vi "Initialize Virtual Microscope.vi"(8 "error in (no error)":errorcluster, 11 "Application in":refnum<class "Application.lvclass">) -> (0 "error out":errorcluster, 3 "Application out":refnum<class "Application.lvclass">)   [LabVIEW 2023, in "Application.lvlib" / "Application.lvclass"]
uses:
  Application.lvclass
  Application.lvclass/Application.ctl
  <vilib>/ActorFramework/Actor/Actor.lvclass
  User Interface/Splash Screen Messages/Update Status Msg/Update Status Msg.lvclass
  Hardware/Microscope/Microscope.lvclass
  C:/FlashGordon/Development/Hardware/Device/Device.lvclass
  C:/Program Files/National Instruments/LabVIEW 2023/vi.lib/ActorFramework/Actor/Actor.lvclass
  C:/FlashGordon/Development/Hardware/Microscope/Microscope.lvclass
  C:/FlashGordon/Development/Application/Application.lvclass
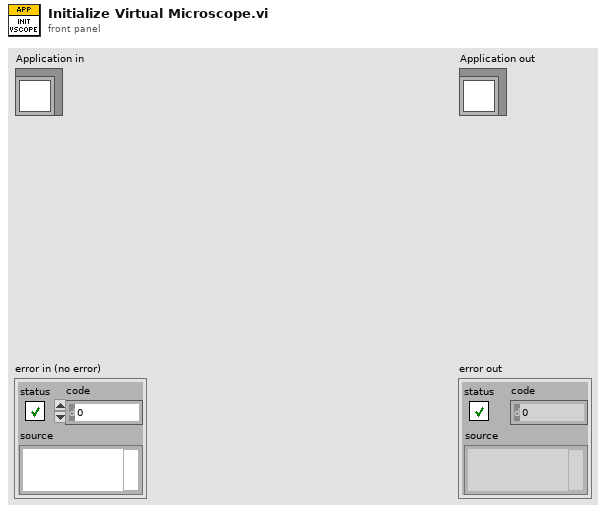
[diagram p1: front panel]
types:
  T1 = typedef "Microscope Type.ctl" = enum16{"Disable", "TE2000", "Eclipse Ti", "Ti2"}
  T2 = typedef "Microscope Configuration.ctl" = cluster{"Serial Port":refnum<visa-resource-name>, "Microscope Type":T1, "Detection Settings":cluster{"Name":string, "Filter Position":u16, "Optical Path":u16}[]}
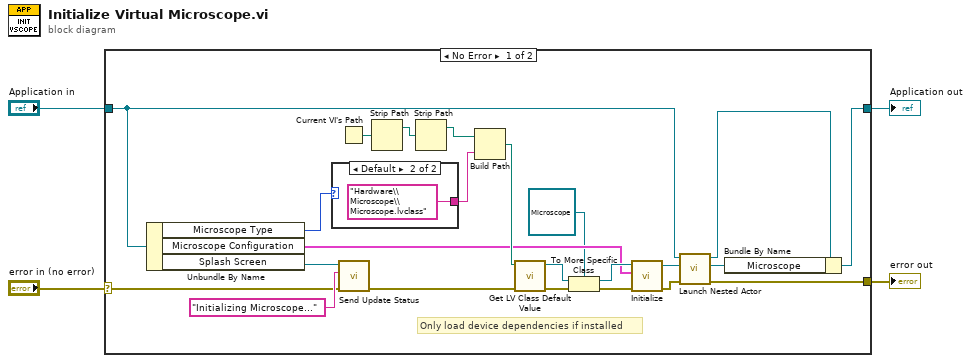
[diagram p0: block diagram]
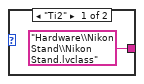
[diagram p2: hidden frame]
diagram:
  n1 = case shown="No Error" "error in (no error)" {
    selector: "error in (no error)" -> [w19 w31]
    tunnel: [w25 w31] -> w3
    tunnel: [w26 w30] -> w1
    tunnel: "Application in" -> [w23 w30]
    frame No Error {
      # "Only load device dependencies if installed"
      n2 = Unbundle By Name(w23) -> ("Microscope Type"=w8:T1, "Microscope Configuration"=w6:T2, "Splash Screen"=w18:refnum<class "Message Enqueuer.lvclass">)
      n3 = case shown="Default" w8 {
        tunnel: ["Hardware\\Nikon Stand\\Nikon Stand.lvclass" "Hardware\\Microscope\\Microscope.lvclass"] -> w14
        frame "Ti2" {
        }
        frame Default {
        }
      }
      n4 = Current VI's Path() -> (path=w13:path)
      n5 = call "Send Update Status.vi"("error in (no error)"=w19, "Status Message"="Initializing Microscope...", "Message Enqueuer"=w18) -> ("error out"=w9:errorcluster)  [unwired: 7 in, 1 out]
      n6 = Strip Path(path=w13) -> (stripped path=w12:path)  [unwired: 1 out]
      n7 = Strip Path(path=w12) -> (stripped path=w11:path)  [unwired: 1 out]
      n8 = Build Path(base path=w11, name or relative path=w14) -> (appended path=w15:path)
      n9 = call <vilib>:"Get LV Class Default Value.vi"("error in (no error)"=w9, "class path"=w15) -> ("error out"=w17:errorcluster, "object"=w16:refnum<class>)  [unwired: 8 in]
      n10 = To More Specific Class(target class=refnum<class "Microscope.lvclass"> refnum ("Microscope.lvlib:Microscope.lvclass"), reference=w16, error in=w17) -> (specific class reference=w7:refnum<class "Microscope.lvclass">, error out=w10:errorcluster)
      n11 = call-dynamic "Initialize.vi"("error in (no error)"=w10, "Microscope Configuration"=w6, "Microscope In"=w7) -> ("error out"=w22:errorcluster, "Microscope out"=w21:refnum<class "Microscope.lvclass">)  [unwired: 7 in]
      n12 = call <vilib>:"Launch Nested Actor.vi"("error in (no error)"=w22, "Nested Actor"=w21, "Caller Actor in"=w23) -> ("error out"=w25:errorcluster, "Nested Actor's Enqueuer"=w27:refnum<class "Message Enqueuer.lvclass">, "Caller Actor out"=w24:refnum<class "Application.lvclass">)  [unwired: 6 in]
      n13 = Bundle By Name(cluster=w24, "Microscope"=w27) -> (w26:refnum<class "Application.lvclass">)
    }
    frame Error {
    }
  }
  "error out" <- w3
  "Application out" <- w1
